vi "EX 9-6 LEDPWM(port) XBOX.vi"() -> ()   [LabVIEW 2011]
doc: "An example that reads a user selectable analog input pin on the Arduino."
uses:
  <vilib>/LabVIEW Interface for Arduino/Type Defs/Board Type.ctl
  <vilib>/LabVIEW Interface for Arduino/Type Defs/Connection Type.ctl
  <vilib>/Utility/inputDevices.llb/closeJoystick.vi
  <vilib>/Utility/inputDevices.llb/joystickAcquire.vi
  <vilib>/LabVIEW Interface for Arduino/LabVIEW Interface for Arduino.lvlib
panel:
  out "PWM":i32
  out "axis info":T1
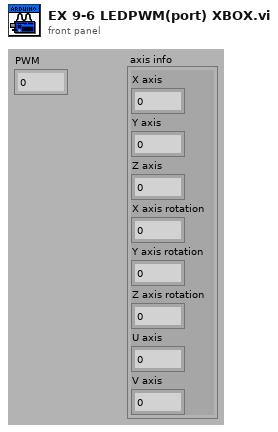
[diagram p1: front panel]
types:
  T1 = cluster{"X axis":i32, "Y axis":i32, "Z axis":i32, "X axis rotation":i32, "Y axis rotation":i32, "Z axis rotation":i32, "U axis":i32, "V axis":i32}
  T2 = typedef "LabVIEW Interface for Arduino.lvlib/Connection Type.ctl" = enum8{"USB / Serial", "XBEE", "BlueSmirf (Bluetooth)"}
  T3 = typedef "LabVIEW Interface for Arduino.lvlib/Board Type.ctl" = enum16{"Uno", "Dimuelanove w/Atmega 328", "Mega 2560"}
  T4 = typedef "LabVIEW Interface for Arduino.lvlib/Arduino Resource.ctl" = cluster{"VISA resource":refnum<visa-resource-name>, "Board Type":T3, "Connection Type":enum8{"USB / Serial"}, "Bytes Per Packet (15)":u8}
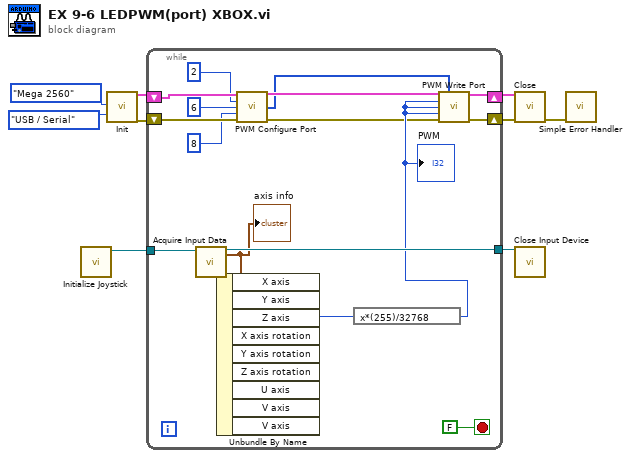
[diagram p0: block diagram]
diagram:
  n1 = call <vilib>:"Initialize Joystick.vi"() -> ("device ID"=w2:refnum<k1>)  [unwired: 10 in, 1 out]
  n2 = call <vilib>:"Init.vi"("Board Type (Uno)"=Board_Type."Mega 2560", "Connection Type (USB/Serial)"=Connection_Type."USB / Serial") -> ("Arduino Resource"=w9:T4, "error out"=w6:errorcluster)  [unwired: 16 in]
  n3 = while {
    shift-right: [w24] -> w8
    shift-left: w9 -> [w17]
    shift-right: [w23] -> w7
    shift-left: w6 -> [w14]
    tunnel: w2 -> [w22]
    tunnel: [w21] -> w1
    stop <- FALSE stop-if-true
    n4 = call-poly <vilib>:"Acquire Input Data.vi"("device ID"=w22) -> ("device ID"=w21:refnum<k1>, "axis info"=w20:T1)  [unwired: 14 in, 3 out]
    "axis info" <- w20
    n5 = Unbundle By Name(w20) -> ("Z axis"=w19:i32)  [unwired: 8 out]
    n6 = call <vilib>:"PWM Configure Port.vi"("Arduino Resource"=w17, "PWM Pin (3)"=u8 2 ("Digital I/O Pin"), "PWM Pin (5)"=u8 6 ("Digital I/O Pin"), "PWM Pin (6)"=u8 8 ("Digital I/O Pin"), "error in"=w14) -> ("Arduino Resource"=w16:T4, "PWM Pins"=w13:u8[], "error out"=w15:errorcluster)  [unwired: 8 in]
    n7 = expression code="x*(255)/32768"(w19) -> (w18:i32)
    "PWM" <- w18
    n8 = call <vilib>:"PWM Write Port.vi"("Arduino Resource"=w16, "PWM Pins"=w13, "PWM 0 (0-255)"=w18, "PWM 1 (0-255)"=w18, "PWM 2 (0-255)"=w18, "error in"=w15) -> ("Arduino Resource"=w24:T4, "error out"=w23:errorcluster)  [unwired: 7 in, 1 out]
  }
  n9 = call <vilib>:"Close.vi"("Arduino Resource"=w8, "error in"=w7) -> ("error out"=w5:errorcluster)  [unwired: 13 in]
  n10 = call-poly <vilib>:"Close Input Device.vi"("device ID"=w1) -> ()  [unwired: 9 in, 1 out]
  n11 = call <vilib>:"Simple Error Handler.vi"("error in (no error)"=w5) -> ()  [unwired: 4 in, 5 out]
